vi "quiz3.vi"() -> ()   [LabVIEW 2017]
uses:
  <vilib>/Utility/file.llb/Read Delimited Spreadsheet (string).vi
panel:
  in  "stop 2":bool
  in  "stop":bool
  out "Tab Control 2":T1(tab)
  in  "Contraseña 2":string
  in  "Login 2":string
  in  "Ingresar 2":bool=TRUE
  in  "Ingrese posicion 2":i32
  in  "Usuario a borrar 2":string
  in  "Agregar 2":bool
  in  "Nuevo usuario 2":string
  in  "Nueva contraseña 2":string
  in  "eliminar 2":bool
  in  "Terminar sesion 3":bool
  out "Usuario 2":string
  in  "Terminar sesion 4":bool
  out "leeradd 2":string[][](array[string])
  out "element 4":string
  out "Usuarios y contraseñas 2":string[](array[string])
  out "element 3":i32
  out "Usuarios 2":string[](array[string])
  out "Usuarios":string[](array[string])
  out "element 2":i32
  out "Usuarios y contraseñas":string[](array[string])
  out "leeradd":string[][](array[string])
  out "element":string
  out "Tab Control":T1(tab)
  in  "Contraseña":string
  in  "Login":string
  in  "Ingresar":bool=TRUE
  in  "Ingrese posicion":i32
  in  "Usuario a borrar":string
  in  "Agregar":bool
  in  "Nuevo usuario":string
  in  "Nueva contraseña":string
  in  "eliminar":bool
  in  "Terminar sesion 2":bool
  out "Usuario":string
  in  "Terminar sesion":bool
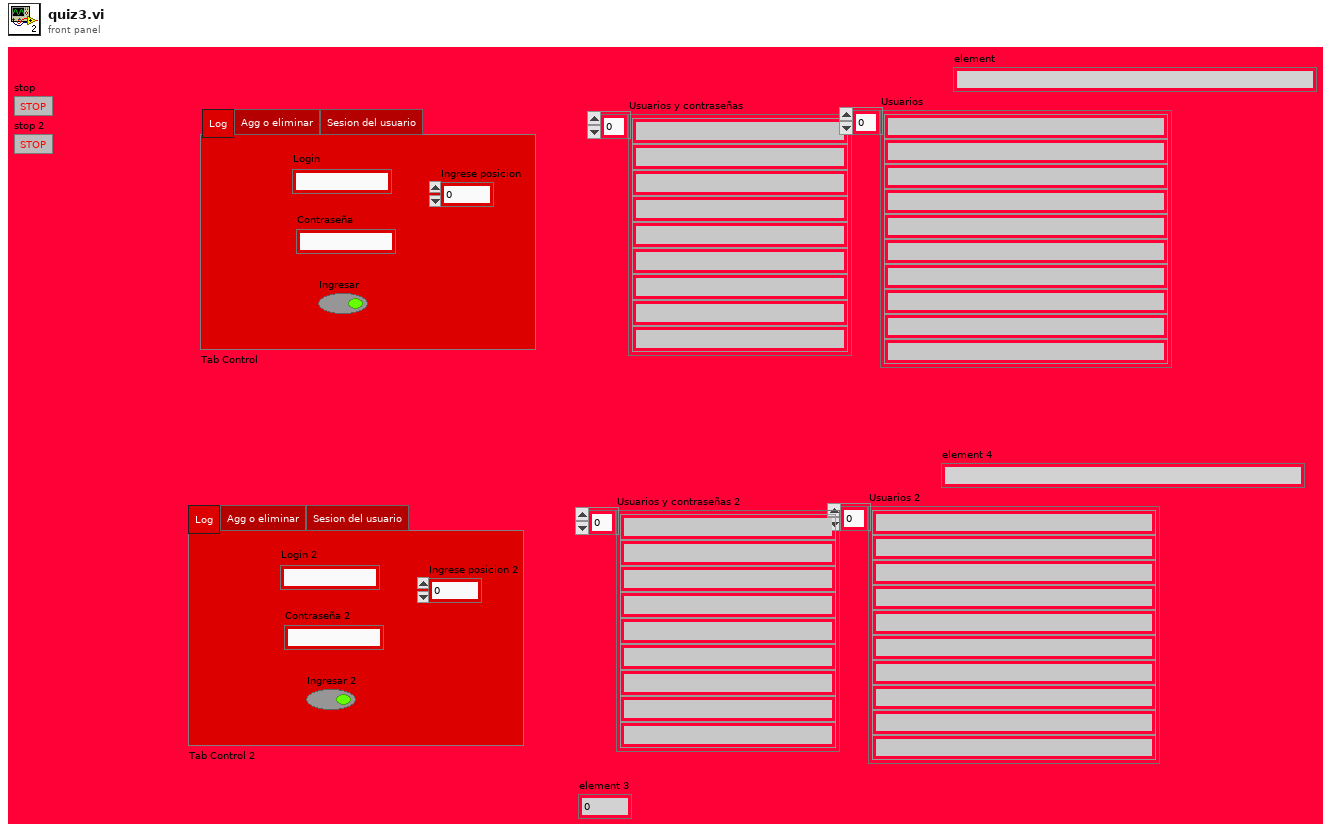
[diagram p1: front panel]
types:
  T1 = enum32{"Log", "Agg o eliminar", "Sesion del usuario"}
  T2 = enum16{"open", "replace", "create", "open or create", "replace or create", "replace or create with confirmation"}
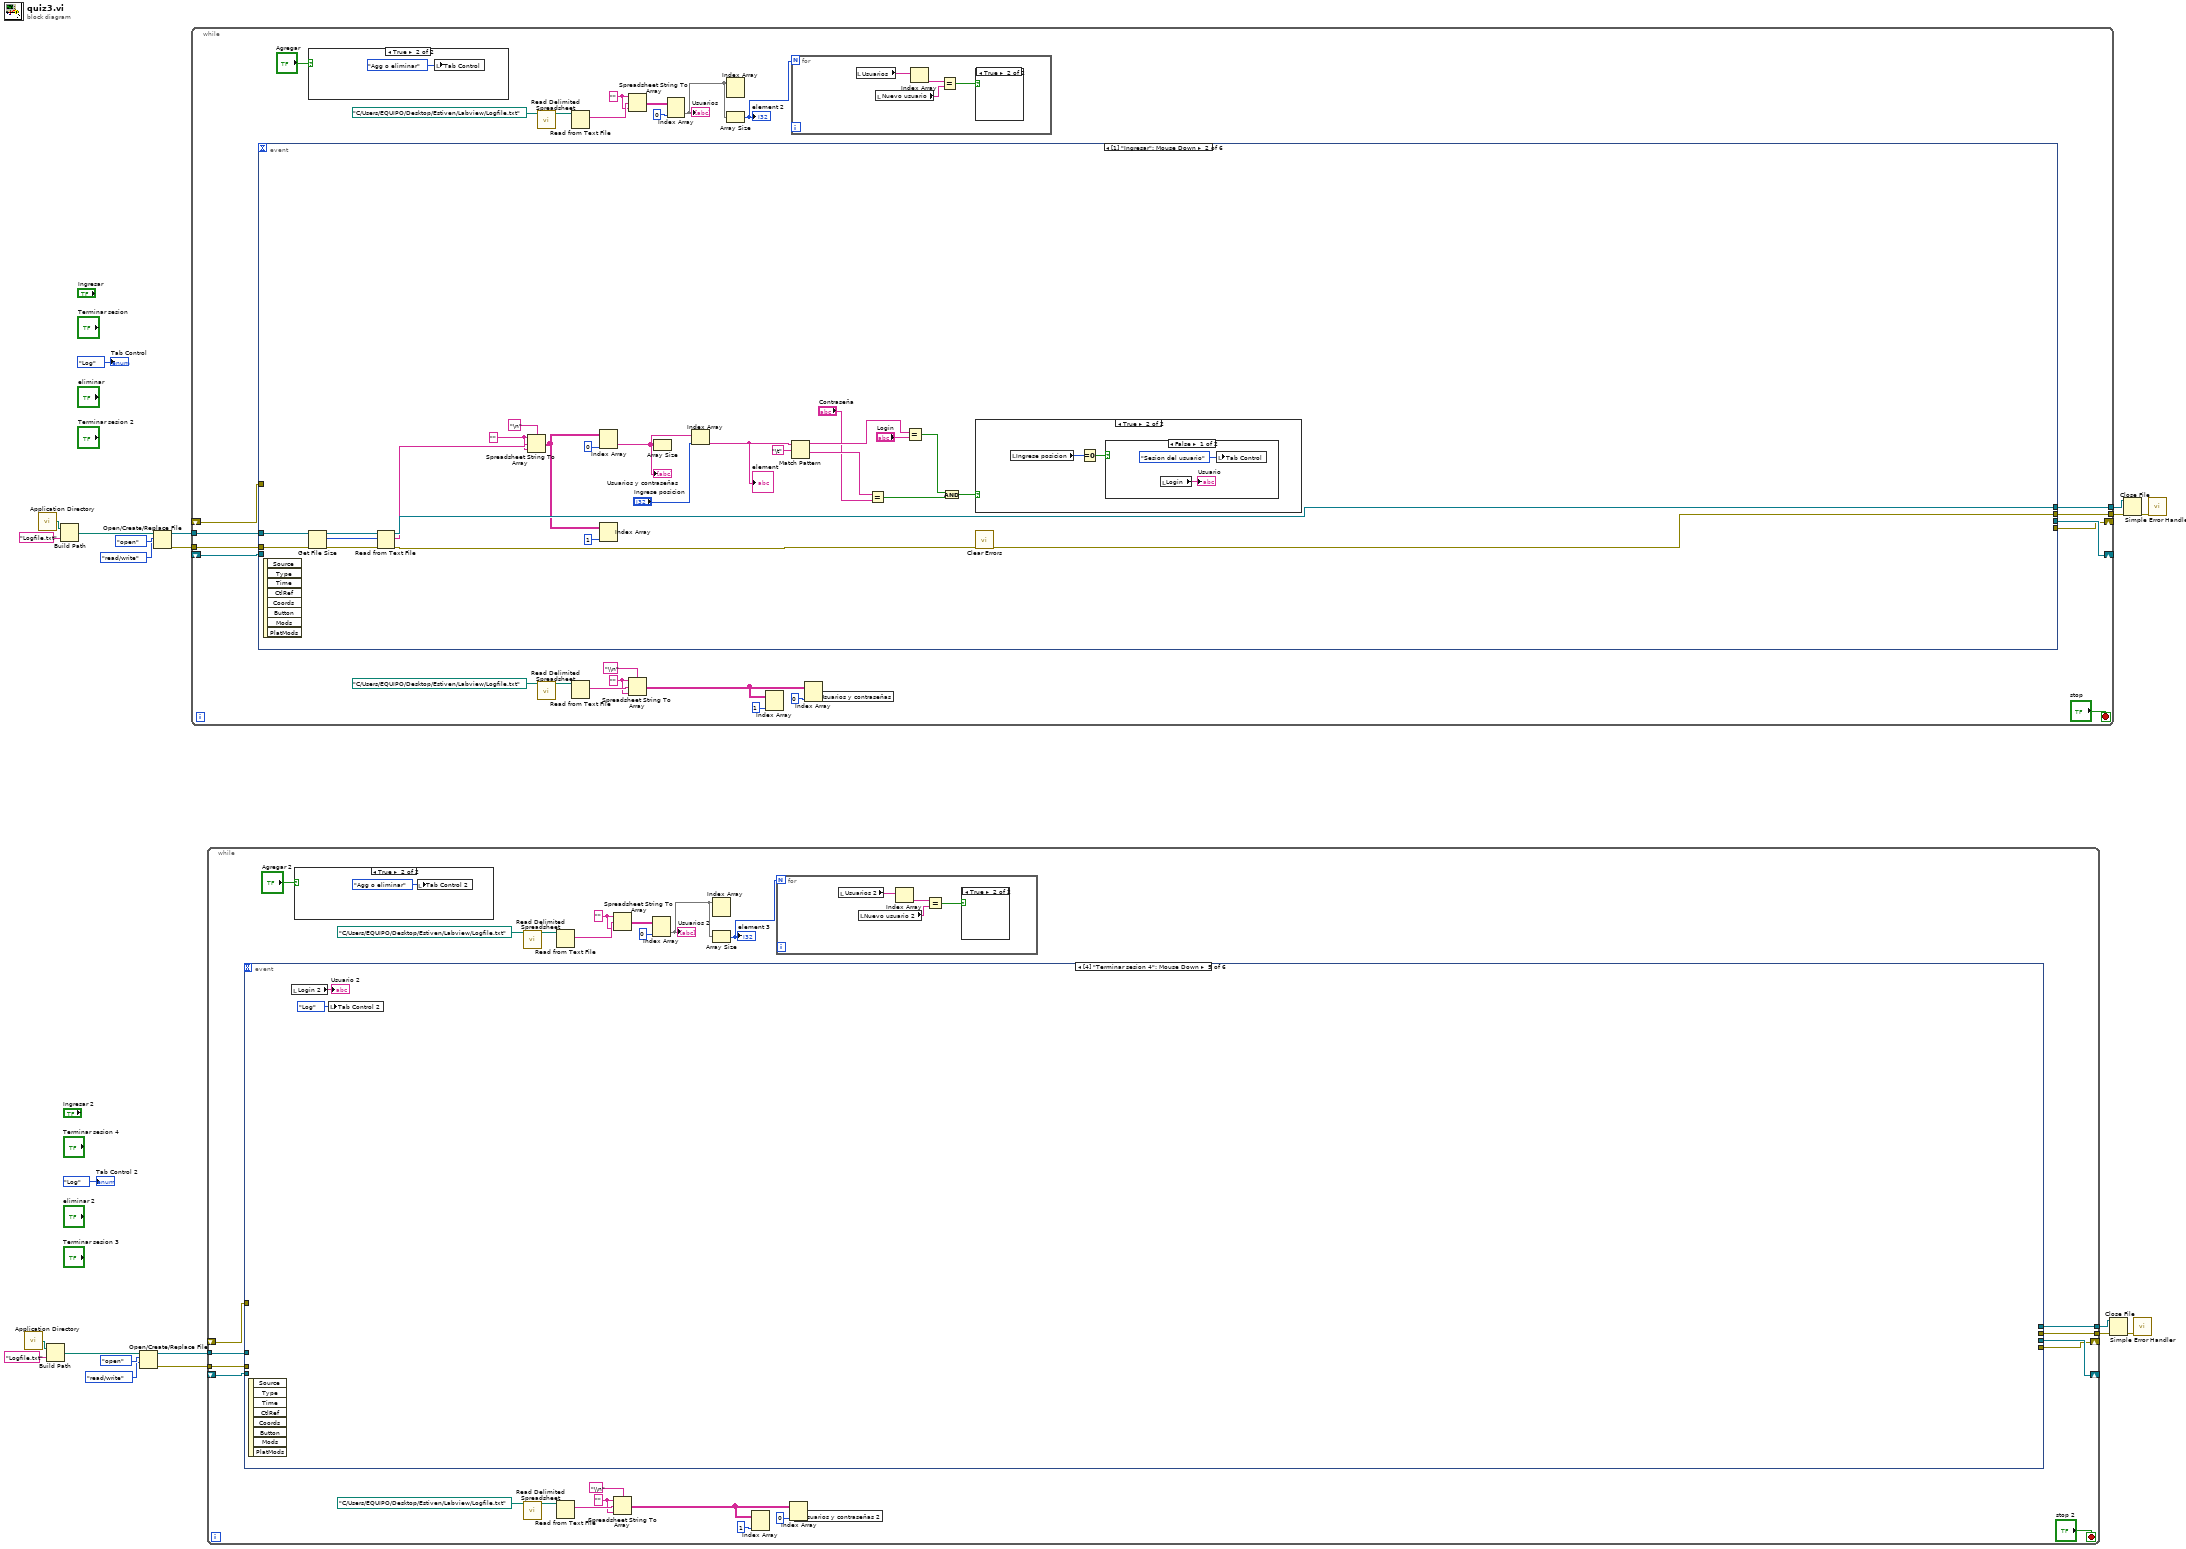
[diagram p0: block diagram]
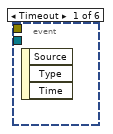
[diagram p4: hidden frame]
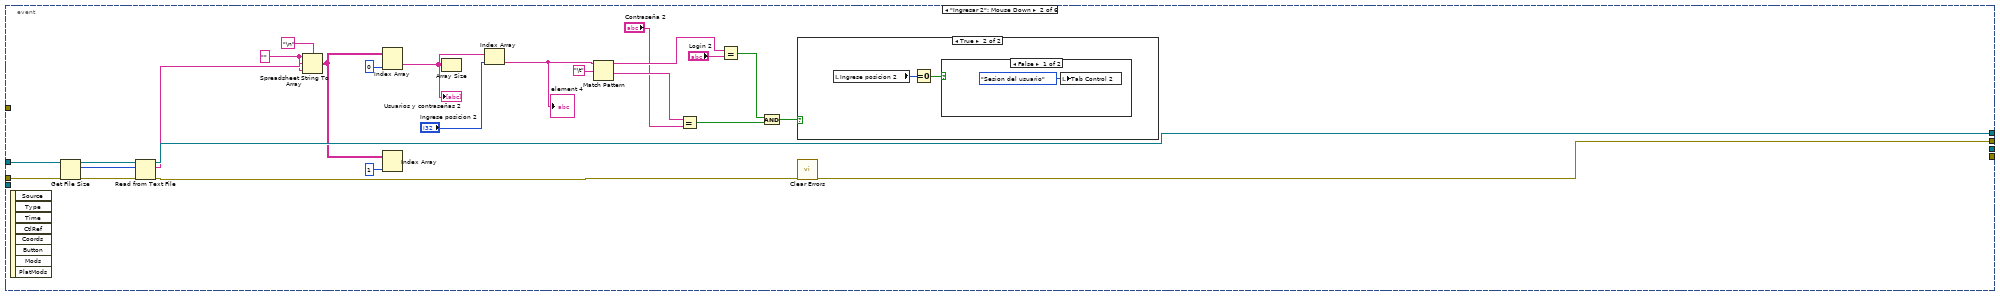
[diagram p5: hidden frame]
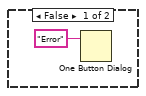
[diagram p6: hidden frame]
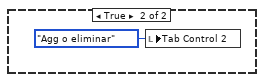
[diagram p7: hidden frame]
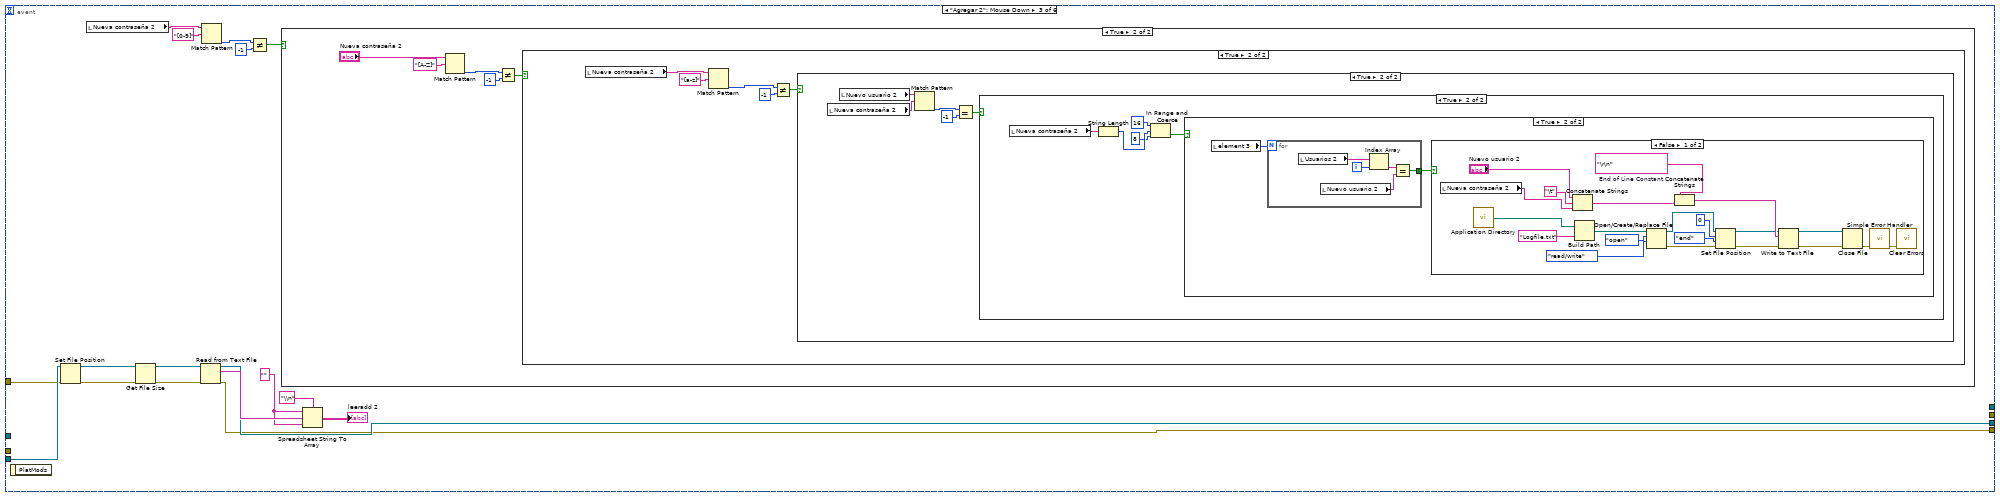
[diagram p8: hidden frame]
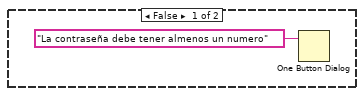
[diagram p9: hidden frame]
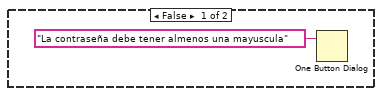
[diagram p10: hidden frame]
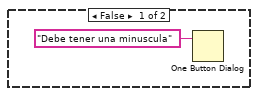
[diagram p11: hidden frame]
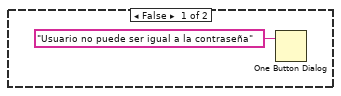
[diagram p12: hidden frame]
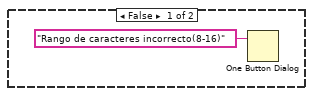
[diagram p13: hidden frame]
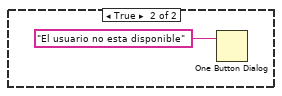
[diagram p14: hidden frame]
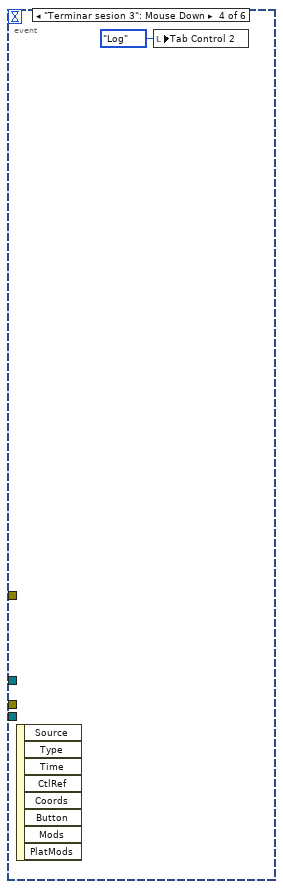
[diagram p15: hidden frame]
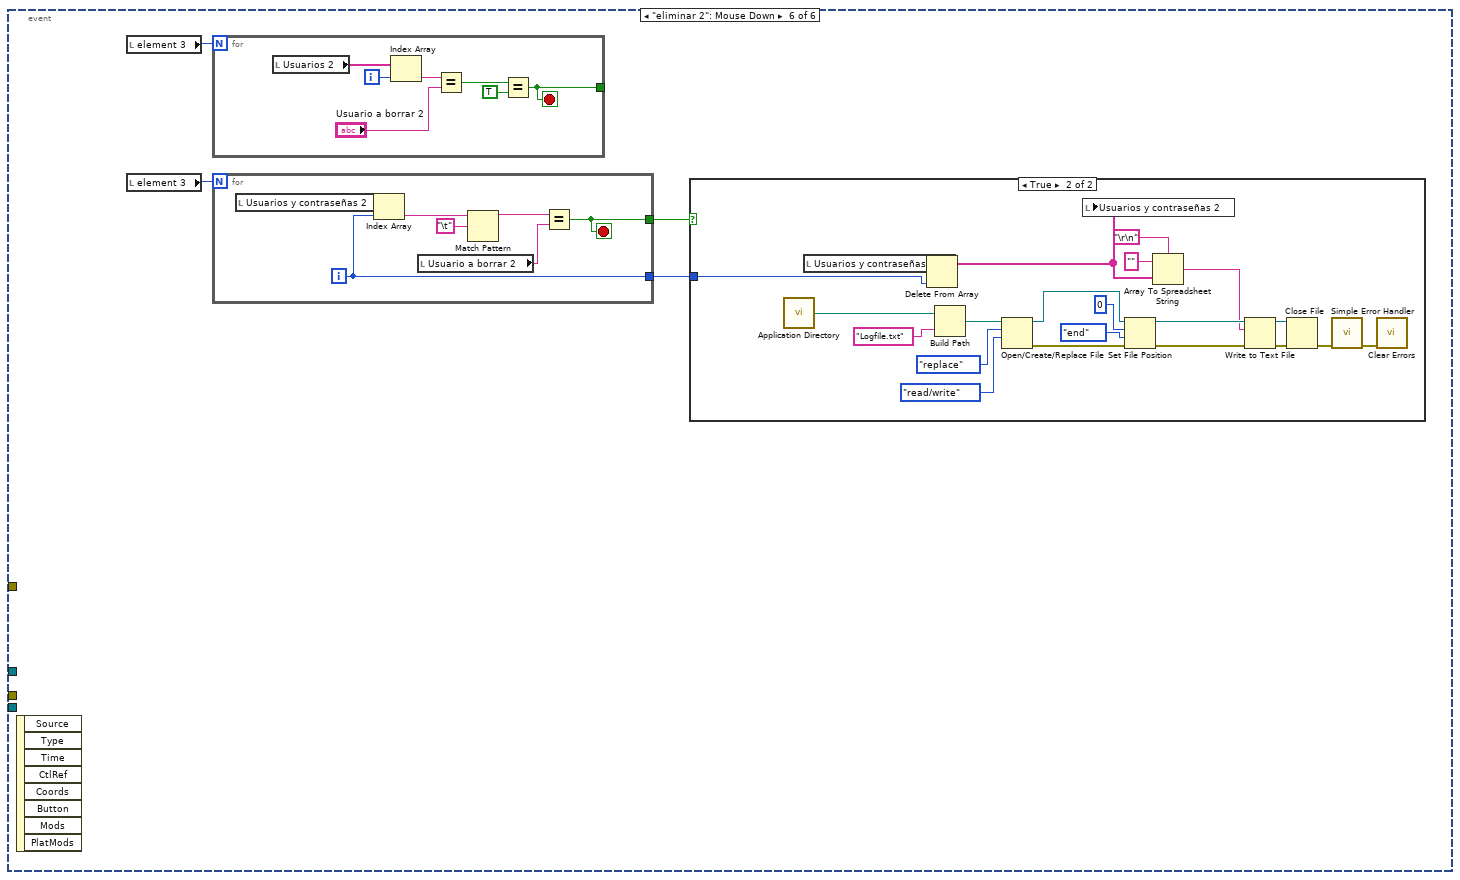
[diagram p16: hidden frame]
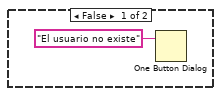
[diagram p17: hidden frame]
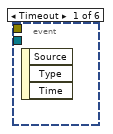
[diagram p20: hidden frame]
diagram:
  n1 = call <vilib>:"Application Directory.vi"() -> ("Application Directory"=w5:path)
  n2 = call <vilib>:"Application Directory.vi"() -> ("Application Directory"=w16:path)
  n3 = Build Path(base path=w5, name or relative path="Logfile.txt") -> (appended path=w6:path)
  n4 = Build Path(base path=w16, name or relative path="Logfile.txt") -> (appended path=w17:path)
  n5 = Open/Create/Replace File(file path (use dialog)=w6, operation (0:open)=T2."open", access (0:read/write)=enum16{"read/write", "read-only", "write-only"}."read/write") -> (refnum out=w8:refnum<file>, error out=w11:errorcluster)  [unwired: 3 in, 1 out]
  n6 = Open/Create/Replace File(file path (use dialog)=w17, operation (0:open)=T2."open", access (0:read/write)=enum16{"read/write", "read-only", "write-only"}."read/write") -> (refnum out=w19:refnum<file>, error out=w22:errorcluster)  [unwired: 3 in, 1 out]
  n7 = while {
    tunnel: w22 -> [w45]
    tunnel: [w49] -> w21
    tunnel: w19 -> [w48]
    tunnel: [w47] -> w18
    shift-right: [w42] -> _
    shift-left: _ -> [w44]
    shift-right: [w41] -> _
    shift-left: _ -> [w43]
    stop <- "stop" stop-if-true
    w26 = "" ("format string")
    w36 = "" ("format string")
    n8 = event shown="[1] \"Ingresar\": Mouse Down" {
      selector: _ -> [_ _ _ _ _ _]
      dyn-events: _ -> [_ _ _ _ _ _]
      timeout: _ -> [_ _ _ _ _ _]
      tunnel: w45 -> [_ w71 _ _ _ _]
      tunnel: [_ w78 _ _ _ _] -> w49
      tunnel: w48 -> [_ w72 _ _ _ _]
      tunnel: [_ w74 _ _ _ _] -> w47
      tunnel: w44 -> [_ _ w90 _ _ _]
      tunnel: w43 -> [_ _ w89 _ _ _]
      tunnel: [_ _ w87 _ _ _] -> w42
      tunnel: [_ _ w86 _ _ _] -> w41
      event Timeout {
        n9 = event-data() -> ()  [unwired: 1 in, 3 out]
      }
      event "Ingresar": Mouse Down {
        w64 = "" ("format string")
        n10 = event-data() -> ()  [unwired: 1 in, 8 out]
        n11 = Get File Size(file=w72, error in=w71) -> (refnum out=w70:refnum<file>, size (in bytes)=w69:i64, 0:w68:errorcluster)
        n12 = Read from Text File(file (use dialog)=w70, count=w69, error in=w68) -> (refnum out=w74:refnum<file>, text=w65:string, error out=w79:errorcluster)  [unwired: 1 in, 1 out]
        n13 = Spreadsheet String To Array(delimiter (Tab)="\n", format string=w64, spreadsheet string=w65, array type (2D Dbl)=w64) -> (array=w63:string[][])
        n14 = Index Array "Index Array"(array=w63, index (col)=0 ("disabled index (col)")) -> (element=w55:string[])  [unwired: 1 in]
        "Usuarios y contraseñas" <- w55
        n15 = Index Array "Index Array"(array=w63, index (col)=1 ("disabled index (col)")) -> ()  [unwired: 1 in, 1 out]
        n16 = Array Size(array=w55) -> ()  [unwired: 1 out]
        n17 = Index Array "Index Array"(array=w55, index="Ingrese posicion") -> (element=w56:string)
        "element" <- w56
        n18 = Match Pattern(string=w56, regular expression="\t") -> (before substring=w67:string, after substring=w66:string)  [unwired: 1 in, 2 out]
        n19 = Equal?(x=w66, y="Contraseña") -> (x = y?=w76:bool)
        n20 = Equal?(x=w67, y="Login") -> (x = y?=w77:bool)
        n21 = And(x=w77, y=w76) -> (x .and. y?=w75:bool)
        n22 = case shown="True" w75 {
          frame False {
            n23 = One Button Dialog(message="Error") -> ()  [unwired: 1 in, 1 out]
          }
          frame True {
            n24 = local read "Ingrese posicion"() -> (w82:i32)
            n25 = Equal To 0?(x=w82) -> (x = 0?=w81:bool)
            n26 = case shown="False" w81 {
              frame False {
                n27 = local read "Login"() -> (→"Usuario":string)
                n28 = local write "Tab Control"(T1."Sesion del usuario" ("Tab Control")) -> ()
              }
              frame True {
                n29 = local write "Tab Control"(enum32{"Log", "Agg o eliminar"}."Agg o eliminar" ("Tab Control")) -> ()
              }
            }
          }
        }
        n30 = call <vilib>:"Clear Errors.vi"("error in (no error)"=w79) -> ("error out"=w78:errorcluster)  [unwired: 5 in, 1 out]
      }
      event "Agregar": Mouse Down {
        w91 = "" ("format string")
        n31 = event-data() -> ()  [unwired: 1 in, 1 out]
        n32 = Set File Position(refnum=w90, error in=w89) -> (refnum out=w97:refnum<file>, error out=w94:errorcluster)  [unwired: 2 in]
        n33 = local read "Nueva contraseña"() -> (w102:string)
        n34 = Get File Size(file=w97, error in=w94) -> (refnum out=w96:refnum<file>, 0:w93:errorcluster)  [unwired: 1 out]
        n35 = Read from Text File(file (use dialog)=w96, error in=w93) -> (refnum out=w87:refnum<file>, text=w95:string, error out=w86:errorcluster)  [unwired: 2 in, 1 out]
        n36 = Match Pattern(string=w102, regular expression="[0-9]") -> (offset past match=w100:i32)  [unwired: 1 in, 3 out]
        n37 = Not Equal?(x=w100, y=-1) -> (x != y?=w98:bool)
        n38 = case shown="True" w98 {
          frame False {
            n39 = One Button Dialog(message="La contraseña debe tener almenos un numero") -> ()  [unwired: 1 in, 1 out]
          }
          frame True {
            n40 = Match Pattern(string="Nueva contraseña", regular expression="[A-Z]") -> (offset past match=w107:i32)  [unwired: 1 in, 3 out]
            n41 = Not Equal?(x=w107, y=-1) -> (x != y?=w104:bool)
            n42 = case shown="True" w104 {
              frame False {
                n43 = One Button Dialog(message="La contraseña debe tener almenos una mayuscula") -> ()  [unwired: 1 in, 1 out]
              }
              frame True {
                n44 = local read "Nueva contraseña"() -> (w111:string)
                n45 = Match Pattern(string=w111, regular expression="[a-z]") -> (offset past match=w113:i32)  [unwired: 1 in, 3 out]
                n46 = Not Equal?(x=w113, y=-1) -> (x != y?=w110:bool)
                n47 = case shown="True" w110 {
                  frame False {
                    n48 = One Button Dialog(message="Debe tener una minuscula") -> ()  [unwired: 1 in, 1 out]
                  }
                  frame True {
                    n49 = local read "Nueva contraseña"() -> (w120:string)
                    n50 = local read "Nuevo usuario"() -> (w119:string)
                    n51 = Match Pattern(string=w119, regular expression=w120) -> (offset past match=w118:i32)  [unwired: 1 in, 3 out]
                    n52 = Equal?(x=w118, y=-1) -> (x = y?=w117:bool)
                    n53 = case shown="True" w117 {
                      frame False {
                        n54 = One Button Dialog(message="Usuario no puede ser igual a la contraseña") -> ()  [unwired: 1 in, 1 out]
                      }
                      frame True {
                        n55 = local read "Nueva contraseña"() -> (w126:string)
                        n56 = String Length(string=w126) -> (length=w125:i32)
                        n57 = In Range and Coerce(upper limit=16, x=w125, lower limit=8) -> (In Range?=w122:bool)  [unwired: 1 out]
                        n58 = case shown="True" w122 {
                          frame False {
                            n59 = One Button Dialog(message="Rango de caracteres incorrecto(8-16)") -> ()  [unwired: 1 in, 1 out]
                          }
                          frame True {
                            n60 = local read "element 2"() -> (w129:i32)
                            n61 = for {
                              N: w129 -> [_]
                              tunnel: [w154] -> w128
                              i -> [w152]
                              n62 = local read "Usuarios"() -> (w153:string[])
                              n63 = local read "Nuevo usuario"() -> (w156:string)
                              n64 = Index Array(array=w153, index=w152) -> (element=w155:string)
                              n65 = Equal?(x=w155, y=w156) -> (x = y?=w154:bool)
                            }
                            n66 = case shown="False" w128 {
                              frame False {
                                w136 = "\r\n"  # End of Line Constant
                                n67 = local read "Nueva contraseña"() -> (w137:string)
                                n68 = call <vilib>:"Application Directory.vi"() -> ("Application Directory"=w139:path)
                                n69 = Concatenate Strings "Concatenate Strings"("Nuevo usuario", "\t", w137) -> (w150:string)
                                n70 = Build Path(base path=w139, name or relative path="Logfile.txt") -> (appended path=w140:path)
                                n71 = Open/Create/Replace File(file path (use dialog)=w140, operation (0:open)=T2."open", access (0:read/write)=enum16{"read/write", "read-only", "write-only"}."read/write") -> (refnum out=w141:refnum<file>, error out=w144:errorcluster)  [unwired: 3 in, 1 out]
                                n72 = Concatenate Strings "Concatenate Strings"(w136, w150) -> (w149:string)
                                n73 = Set File Position(offset (in bytes) (0)=i64 0, refnum=w141, from (0:start)=enum16{"start", "end", "current"}."end", error in=w144) -> (refnum out=w142:refnum<file>, error out=w145:errorcluster)
                                n74 = Write to Text File(file (use dialog)=w142, text=w149, error in=w145) -> (refnum out=w143:refnum<file>, error out=w146:errorcluster)  [unwired: 1 in, 1 out]
                                n75 = Close File(refnum=w143, error in=w146) -> (error out=w147:errorcluster)  [unwired: 1 out]
                                n76 = call <vilib>:"Simple Error Handler.vi"("error in (no error)"=w147) -> ("error out"=w148:errorcluster)  [unwired: 4 in, 4 out]
                                n77 = call <vilib>:"Clear Errors.vi"("error in (no error)"=w148) -> ()  [unwired: 5 in, 2 out]
                              }
                              frame True {
                                n78 = One Button Dialog(message="El usuario no esta disponible") -> ()  [unwired: 1 in, 1 out]
                              }
                            }
                          }
                        }
                      }
                    }
                  }
                }
              }
            }
          }
        }
        n79 = Spreadsheet String To Array(delimiter (Tab)="\\n", format string=w91, spreadsheet string=w95, array type (2D Dbl)=w91) -> (array=→"leeradd":string[][])
      }
      event "Terminar sesion 2": Mouse Down {
        n80 = event-data() -> ()  [unwired: 1 in, 8 out]
        n81 = local write "Tab Control"(T1."Log" ("Tab Control")) -> ()
      }
      event "Terminar sesion": Mouse Down {
        n82 = event-data() -> ()  [unwired: 1 in, 8 out]
        n83 = local write "Tab Control"(T1."Log" ("Tab Control")) -> ()
      }
      event "eliminar": Mouse Down {
        n84 = event-data() -> ()  [unwired: 1 in, 8 out]
        n85 = local read "element 2"() -> (w162:i32)
        n86 = local read "element 2"() -> (w161:i32)
        n87 = for {
          N: w162 -> [_]
          tunnel: [w171] -> _
          i -> [w170]
          stop <- w171 stop-if-true
          n88 = local read "Usuarios"() -> (w173:string[])
          n89 = Index Array(array=w173, index=w170) -> (element=w172:string)
          n90 = Equal?(x=w172, y="Usuario a borrar") -> (x = y?=w176:bool)
          n91 = Equal?(x=w176, y=TRUE) -> (x = y?=w171:bool)
        }
        n92 = for {
          N: w161 -> [_]
          tunnel: [w165] -> w159
          tunnel: [w163] -> w160
          i -> [w163]
          stop <- w165 stop-if-true
          n93 = local read "Usuarios y contraseñas"() -> (w164:string[])
          n94 = Index Array(array=w164, index=w163) -> (element=w169:string)
          n95 = local read "Usuario a borrar"() -> (w166:string)
          n96 = Match Pattern(string=w169, regular expression="\t") -> (before substring=w167:string)  [unwired: 1 in, 3 out]
          n97 = Equal?(x=w167, y=w166) -> (x = y?=w165:bool)
        }
        n98 = case shown="True" w159 {
          tunnel: w160 -> [_ w183]
          frame False {
            n99 = One Button Dialog(message="El usuario no existe") -> ()  [unwired: 1 in, 1 out]
          }
          frame True {
            n100 = call <vilib>:"Application Directory.vi"() -> ("Application Directory"=w189:path)
            n101 = local read "Usuarios y contraseñas"() -> (w182:string[])
            n102 = Delete From Array "Delete From Array"(array=w182, index=w183) -> (array with subset deleted=w180:string[])  [unwired: 1 in, 1 out]
            n103 = Build Path(base path=w189, name or relative path="Logfile.txt") -> (appended path=w190:path)
            n104 = Open/Create/Replace File(file path (use dialog)=w190, operation (0:open)=T2."replace", access (0:read/write)=enum16{"read/write", "read-only", "write-only"}."read/write") -> (refnum out=w191:refnum<file>, error out=w194:errorcluster)  [unwired: 3 in, 1 out]
            n105 = local write "Usuarios y contraseñas"(w180) -> ()
            n106 = Set File Position(offset (in bytes) (0)=i64 0, refnum=w191, from (0:start)=enum16{"start", "end", "current"}."end", error in=w194) -> (refnum out=w192:refnum<file>, error out=w195:errorcluster)
            n107 = Array To Spreadsheet String(delimiter (Tab)="\r\n", array=w180, 3:"" ("format string")) -> (spreadsheet string=w179:string)
            n108 = Write to Text File(file (use dialog)=w192, text=w179, error in=w195) -> (refnum out=w193:refnum<file>, error out=w196:errorcluster)  [unwired: 1 in, 1 out]
            n109 = Close File(refnum=w193, error in=w196) -> (error out=w197:errorcluster)  [unwired: 1 out]
            n110 = call <vilib>:"Simple Error Handler.vi"("error in (no error)"=w197) -> ("error out"=w198:errorcluster)  [unwired: 4 in, 4 out]
            n111 = call <vilib>:"Clear Errors.vi"("error in (no error)"=w198) -> ()  [unwired: 5 in, 2 out]
          }
        }
      }
    }
    n112 = case shown="True" "Agregar" {
      frame False {
      }
      frame True {
        n113 = local write "Tab Control"(T1."Agg o eliminar" ("Tab Control")) -> ()
      }
    }
    n114 = call-poly <vilib>:"Read Delimited Spreadsheet.vi"("file path (dialog if empty)"=path "C:/Users/EQUIPO/Desktop/Estiven/Labview/Logfile.txt") -> ("new file path (Not A Path if cancelled)"=w37:path)  [unwired: 9 in, 5 out]
    n115 = call-poly <vilib>:"Read Delimited Spreadsheet.vi"("file path (dialog if empty)"=path "C:/Users/EQUIPO/Desktop/Estiven/Labview/Logfile.txt") -> ("new file path (Not A Path if cancelled)"=w32:path)  [unwired: 9 in, 5 out]
    n116 = Read from Text File(file (use dialog)=w37) -> (text=w38:string)  [unwired: 3 in, 3 out]
    n117 = Read from Text File(file (use dialog)=w32) -> (text=w31:string)  [unwired: 3 in, 3 out]
    n118 = Spreadsheet String To Array(format string=w36, spreadsheet string=w38, array type (2D Dbl)=w36) -> (array=w39:string[][])  [unwired: 1 in]
    n119 = Spreadsheet String To Array(delimiter (Tab)="\\n", format string=w26, spreadsheet string=w31, array type (2D Dbl)=w26) -> (array=w30:string[][])
    n120 = Index Array(array=w39, index (col)=0 ("index")) -> (element=w33:string[])  [unwired: 1 in]
    "Usuarios" <- w33
    n121 = Index Array "Index Array"(array=w33) -> ()  [unwired: 2 in, 2 out]
    n122 = Array Size(array=w33) -> (size(s)=w40:i32)
    "element 2" <- w40
    n123 = Index Array(array=w30, index (col)=1 ("disabled index (col)")) -> ()  [unwired: 1 in, 1 out]
    n124 = for {
      N: w40 -> [_]
      n125 = local read "Usuarios"() -> (w53:string[])
      n126 = local read "Nuevo usuario"() -> (w51:string)
      n127 = Index Array(array=w53) -> (element=w52:string)  [unwired: 1 in]
      n128 = Equal?(x=w52, y=w51) -> (x = y?=w50:bool)
      n129 = case shown="True" w50 {
        frame False {
        }
        frame True {
        }
      }
    }
    n130 = Index Array(array=w30, index (col)=0 ("index")) -> (element=w29:string[])  [unwired: 1 in]
    n131 = local write "Usuarios y contraseñas"(w29) -> ()
  }
  n132 = while {
    tunnel: w11 -> [w221]
    tunnel: [w225] -> w10
    tunnel: w8 -> [w224]
    tunnel: [w223] -> w7
    shift-right: [w218] -> _
    shift-left: _ -> [w220]
    shift-right: [w217] -> _
    shift-left: _ -> [w219]
    stop <- "stop 2" stop-if-true
    w202 = "" ("format string")
    w212 = "" ("format string")
    n133 = event shown="[4] \"Terminar sesion 4\": Mouse Down" {
      selector: _ -> [_ _ _ _ _ _]
      dyn-events: _ -> [_ _ _ _ _ _]
      timeout: _ -> [_ _ _ _ _ _]
      tunnel: w221 -> [_ w247 _ _ _ _]
      tunnel: [_ w254 _ _ _ _] -> w225
      tunnel: w224 -> [_ w248 _ _ _ _]
      tunnel: [_ w250 _ _ _ _] -> w223
      tunnel: w220 -> [_ _ w265 _ _ _]
      tunnel: w219 -> [_ _ w264 _ _ _]
      tunnel: [_ _ w262 _ _ _] -> w218
      tunnel: [_ _ w261 _ _ _] -> w217
      event Timeout {
        n134 = event-data() -> ()  [unwired: 1 in, 3 out]
      }
      event "Ingresar 2": Mouse Down {
        w240 = "" ("format string")
        n135 = event-data() -> ()  [unwired: 1 in, 8 out]
        n136 = Get File Size(file=w248, error in=w247) -> (refnum out=w246:refnum<file>, size (in bytes)=w245:i64, 0:w244:errorcluster)
        n137 = Read from Text File(file (use dialog)=w246, count=w245, error in=w244) -> (refnum out=w250:refnum<file>, text=w241:string, error out=w255:errorcluster)  [unwired: 1 in, 1 out]
        n138 = Spreadsheet String To Array(delimiter (Tab)="\n", format string=w240, spreadsheet string=w241, array type (2D Dbl)=w240) -> (array=w239:string[][])
        n139 = Index Array "Index Array"(array=w239, index (col)=0 ("disabled index (col)")) -> (element=w231:string[])  [unwired: 1 in]
        "Usuarios y contraseñas 2" <- w231
        n140 = Index Array "Index Array"(array=w239, index (col)=1 ("disabled index (col)")) -> ()  [unwired: 1 in, 1 out]
        n141 = Array Size(array=w231) -> ()  [unwired: 1 out]
        n142 = Index Array "Index Array"(array=w231, index="Ingrese posicion 2") -> (element=w232:string)
        "element 4" <- w232
        n143 = Match Pattern(string=w232, regular expression="\t") -> (before substring=w243:string, after substring=w242:string)  [unwired: 1 in, 2 out]
        n144 = Equal?(x=w242, y="Contraseña 2") -> (x = y?=w252:bool)
        n145 = Equal?(x=w243, y="Login 2") -> (x = y?=w253:bool)
        n146 = And(x=w253, y=w252) -> (x .and. y?=w251:bool)
        n147 = case shown="True" w251 {
          frame False {
            n148 = One Button Dialog(message="Error") -> ()  [unwired: 1 in, 1 out]
          }
          frame True {
            n149 = local read "Ingrese posicion 2"() -> (w258:i32)
            n150 = Equal To 0?(x=w258) -> (x = 0?=w257:bool)
            n151 = case shown="False" w257 {
              frame False {
                n152 = local write "Tab Control 2"(T1."Sesion del usuario" ("Tab Control")) -> ()
              }
              frame True {
                n153 = local write "Tab Control 2"(enum32{"Log", "Agg o eliminar"}."Agg o eliminar" ("Tab Control")) -> ()
              }
            }
          }
        }
        n154 = call <vilib>:"Clear Errors.vi"("error in (no error)"=w255) -> ("error out"=w254:errorcluster)  [unwired: 5 in, 1 out]
      }
      event "Agregar 2": Mouse Down {
        w266 = "" ("format string")
        n155 = event-data() -> ()  [unwired: 1 in, 1 out]
        n156 = Set File Position(refnum=w265, error in=w264) -> (refnum out=w272:refnum<file>, error out=w269:errorcluster)  [unwired: 2 in]
        n157 = local read "Nueva contraseña 2"() -> (w277:string)
        n158 = Get File Size(file=w272, error in=w269) -> (refnum out=w271:refnum<file>, 0:w268:errorcluster)  [unwired: 1 out]
        n159 = Read from Text File(file (use dialog)=w271, error in=w268) -> (refnum out=w262:refnum<file>, text=w270:string, error out=w261:errorcluster)  [unwired: 2 in, 1 out]
        n160 = Match Pattern(string=w277, regular expression="[0-9]") -> (offset past match=w275:i32)  [unwired: 1 in, 3 out]
        n161 = Not Equal?(x=w275, y=-1) -> (x != y?=w273:bool)
        n162 = case shown="True" w273 {
          frame False {
            n163 = One Button Dialog(message="La contraseña debe tener almenos un numero") -> ()  [unwired: 1 in, 1 out]
          }
          frame True {
            n164 = Match Pattern(string="Nueva contraseña 2", regular expression="[A-Z]") -> (offset past match=w282:i32)  [unwired: 1 in, 3 out]
            n165 = Not Equal?(x=w282, y=-1) -> (x != y?=w279:bool)
            n166 = case shown="True" w279 {
              frame False {
                n167 = One Button Dialog(message="La contraseña debe tener almenos una mayuscula") -> ()  [unwired: 1 in, 1 out]
              }
              frame True {
                n168 = local read "Nueva contraseña 2"() -> (w286:string)
                n169 = Match Pattern(string=w286, regular expression="[a-z]") -> (offset past match=w288:i32)  [unwired: 1 in, 3 out]
                n170 = Not Equal?(x=w288, y=-1) -> (x != y?=w285:bool)
                n171 = case shown="True" w285 {
                  frame False {
                    n172 = One Button Dialog(message="Debe tener una minuscula") -> ()  [unwired: 1 in, 1 out]
                  }
                  frame True {
                    n173 = local read "Nueva contraseña 2"() -> (w295:string)
                    n174 = local read "Nuevo usuario 2"() -> (w294:string)
                    n175 = Match Pattern(string=w294, regular expression=w295) -> (offset past match=w293:i32)  [unwired: 1 in, 3 out]
                    n176 = Equal?(x=w293, y=-1) -> (x = y?=w292:bool)
                    n177 = case shown="True" w292 {
                      frame False {
                        n178 = One Button Dialog(message="Usuario no puede ser igual a la contraseña") -> ()  [unwired: 1 in, 1 out]
                      }
                      frame True {
                        n179 = local read "Nueva contraseña 2"() -> (w301:string)
                        n180 = String Length(string=w301) -> (length=w300:i32)
                        n181 = In Range and Coerce(upper limit=16, x=w300, lower limit=8) -> (In Range?=w297:bool)  [unwired: 1 out]
                        n182 = case shown="True" w297 {
                          frame False {
                            n183 = One Button Dialog(message="Rango de caracteres incorrecto(8-16)") -> ()  [unwired: 1 in, 1 out]
                          }
                          frame True {
                            n184 = local read "element 3"() -> (w304:i32)
                            n185 = for {
                              N: w304 -> [_]
                              tunnel: [w329] -> w303
                              i -> [w327]
                              n186 = local read "Usuarios 2"() -> (w328:string[])
                              n187 = local read "Nuevo usuario 2"() -> (w331:string)
                              n188 = Index Array(array=w328, index=w327) -> (element=w330:string)
                              n189 = Equal?(x=w330, y=w331) -> (x = y?=w329:bool)
                            }
                            n190 = case shown="False" w303 {
                              frame False {
                                w311 = "\r\n"  # End of Line Constant
                                n191 = local read "Nueva contraseña 2"() -> (w312:string)
                                n192 = call <vilib>:"Application Directory.vi"() -> ("Application Directory"=w314:path)
                                n193 = Concatenate Strings "Concatenate Strings"("Nuevo usuario 2", "\t", w312) -> (w325:string)
                                n194 = Build Path(base path=w314, name or relative path="Logfile.txt") -> (appended path=w315:path)
                                n195 = Open/Create/Replace File(file path (use dialog)=w315, operation (0:open)=T2."open", access (0:read/write)=enum16{"read/write", "read-only", "write-only"}."read/write") -> (refnum out=w316:refnum<file>, error out=w319:errorcluster)  [unwired: 3 in, 1 out]
                                n196 = Concatenate Strings "Concatenate Strings"(w311, w325) -> (w324:string)
                                n197 = Set File Position(offset (in bytes) (0)=i64 0, refnum=w316, from (0:start)=enum16{"start", "end", "current"}."end", error in=w319) -> (refnum out=w317:refnum<file>, error out=w320:errorcluster)
                                n198 = Write to Text File(file (use dialog)=w317, text=w324, error in=w320) -> (refnum out=w318:refnum<file>, error out=w321:errorcluster)  [unwired: 1 in, 1 out]
                                n199 = Close File(refnum=w318, error in=w321) -> (error out=w322:errorcluster)  [unwired: 1 out]
                                n200 = call <vilib>:"Simple Error Handler.vi"("error in (no error)"=w322) -> ("error out"=w323:errorcluster)  [unwired: 4 in, 4 out]
                                n201 = call <vilib>:"Clear Errors.vi"("error in (no error)"=w323) -> ()  [unwired: 5 in, 2 out]
                              }
                              frame True {
                                n202 = One Button Dialog(message="El usuario no esta disponible") -> ()  [unwired: 1 in, 1 out]
                              }
                            }
                          }
                        }
                      }
                    }
                  }
                }
              }
            }
          }
        }
        n203 = Spreadsheet String To Array(delimiter (Tab)="\\n", format string=w266, spreadsheet string=w270, array type (2D Dbl)=w266) -> (array=→"leeradd 2":string[][])
      }
      event "Terminar sesion 3": Mouse Down {
        n204 = event-data() -> ()  [unwired: 1 in, 8 out]
        n205 = local write "Tab Control 2"(T1."Log" ("Tab Control")) -> ()
      }
      event "Terminar sesion 4": Mouse Down {
        n206 = event-data() -> ()  [unwired: 1 in, 8 out]
        n207 = local read "Login 2"() -> (→"Usuario 2":string)
        n208 = local write "Tab Control 2"(T1."Log" ("Tab Control")) -> ()
      }
      event "eliminar 2": Mouse Down {
        n209 = event-data() -> ()  [unwired: 1 in, 8 out]
        n210 = local read "element 3"() -> (w338:i32)
        n211 = local read "element 3"() -> (w337:i32)
        n212 = for {
          N: w338 -> [_]
          tunnel: [w347] -> _
          i -> [w346]
          stop <- w347 stop-if-true
          n213 = local read "Usuarios 2"() -> (w349:string[])
          n214 = Index Array(array=w349, index=w346) -> (element=w348:string)
          n215 = Equal?(x=w348, y="Usuario a borrar 2") -> (x = y?=w352:bool)
          n216 = Equal?(x=w352, y=TRUE) -> (x = y?=w347:bool)
        }
        n217 = for {
          N: w337 -> [_]
          tunnel: [w341] -> w335
          tunnel: [w339] -> w336
          i -> [w339]
          stop <- w341 stop-if-true
          n218 = local read "Usuarios y contraseñas 2"() -> (w340:string[])
          n219 = Index Array(array=w340, index=w339) -> (element=w345:string)
          n220 = local read "Usuario a borrar 2"() -> (w342:string)
          n221 = Match Pattern(string=w345, regular expression="\t") -> (before substring=w343:string)  [unwired: 1 in, 3 out]
          n222 = Equal?(x=w343, y=w342) -> (x = y?=w341:bool)
        }
        n223 = case shown="True" w335 {
          tunnel: w336 -> [_ w359]
          frame False {
            n224 = One Button Dialog(message="El usuario no existe") -> ()  [unwired: 1 in, 1 out]
          }
          frame True {
            n225 = call <vilib>:"Application Directory.vi"() -> ("Application Directory"=w365:path)
            n226 = local read "Usuarios y contraseñas 2"() -> (w358:string[])
            n227 = Delete From Array "Delete From Array"(array=w358, index=w359) -> (array with subset deleted=w356:string[])  [unwired: 1 in, 1 out]
            n228 = Build Path(base path=w365, name or relative path="Logfile.txt") -> (appended path=w366:path)
            n229 = Open/Create/Replace File(file path (use dialog)=w366, operation (0:open)=T2."replace", access (0:read/write)=enum16{"read/write", "read-only", "write-only"}."read/write") -> (refnum out=w367:refnum<file>, error out=w370:errorcluster)  [unwired: 3 in, 1 out]
            n230 = local write "Usuarios y contraseñas 2"(w356) -> ()
            n231 = Set File Position(offset (in bytes) (0)=i64 0, refnum=w367, from (0:start)=enum16{"start", "end", "current"}."end", error in=w370) -> (refnum out=w368:refnum<file>, error out=w371:errorcluster)
            n232 = Array To Spreadsheet String(delimiter (Tab)="\r\n", array=w356, 3:"" ("format string")) -> (spreadsheet string=w355:string)
            n233 = Write to Text File(file (use dialog)=w368, text=w355, error in=w371) -> (refnum out=w369:refnum<file>, error out=w372:errorcluster)  [unwired: 1 in, 1 out]
            n234 = Close File(refnum=w369, error in=w372) -> (error out=w373:errorcluster)  [unwired: 1 out]
            n235 = call <vilib>:"Simple Error Handler.vi"("error in (no error)"=w373) -> ("error out"=w374:errorcluster)  [unwired: 4 in, 4 out]
            n236 = call <vilib>:"Clear Errors.vi"("error in (no error)"=w374) -> ()  [unwired: 5 in, 2 out]
          }
        }
      }
    }
    n237 = case shown="True" "Agregar 2" {
      frame False {
      }
      frame True {
        n238 = local write "Tab Control 2"(T1."Agg o eliminar" ("Tab Control")) -> ()
      }
    }
    n239 = call-poly <vilib>:"Read Delimited Spreadsheet.vi"("file path (dialog if empty)"=path "C:/Users/EQUIPO/Desktop/Estiven/Labview/Logfile.txt") -> ("new file path (Not A Path if cancelled)"=w213:path)  [unwired: 9 in, 5 out]
    n240 = call-poly <vilib>:"Read Delimited Spreadsheet.vi"("file path (dialog if empty)"=path "C:/Users/EQUIPO/Desktop/Estiven/Labview/Logfile.txt") -> ("new file path (Not A Path if cancelled)"=w208:path)  [unwired: 9 in, 5 out]
    n241 = Read from Text File(file (use dialog)=w213) -> (text=w214:string)  [unwired: 3 in, 3 out]
    n242 = Read from Text File(file (use dialog)=w208) -> (text=w207:string)  [unwired: 3 in, 3 out]
    n243 = Spreadsheet String To Array(format string=w212, spreadsheet string=w214, array type (2D Dbl)=w212) -> (array=w215:string[][])  [unwired: 1 in]
    n244 = Spreadsheet String To Array(delimiter (Tab)="\\n", format string=w202, spreadsheet string=w207, array type (2D Dbl)=w202) -> (array=w206:string[][])
    n245 = Index Array(array=w215, index (col)=0 ("index")) -> (element=w209:string[])  [unwired: 1 in]
    "Usuarios 2" <- w209
    n246 = Index Array "Index Array"(array=w209) -> ()  [unwired: 2 in, 2 out]
    n247 = Array Size(array=w209) -> (size(s)=w216:i32)
    "element 3" <- w216
    n248 = Index Array(array=w206, index (col)=1 ("disabled index (col)")) -> ()  [unwired: 1 in, 1 out]
    n249 = for {
      N: w216 -> [_]
      n250 = local read "Usuarios 2"() -> (w229:string[])
      n251 = local read "Nuevo usuario 2"() -> (w227:string)
      n252 = Index Array(array=w229) -> (element=w228:string)  [unwired: 1 in]
      n253 = Equal?(x=w228, y=w227) -> (x = y?=w226:bool)
      n254 = case shown="True" w226 {
        frame False {
        }
        frame True {
        }
      }
    }
    n255 = Index Array(array=w206, index (col)=0 ("index")) -> (element=w205:string[])  [unwired: 1 in]
    n256 = local write "Usuarios y contraseñas 2"(w205) -> ()
  }
  n257 = Close File(refnum=w7, error in=w10) -> (error out=w9:errorcluster)  [unwired: 1 out]
  n258 = Close File(refnum=w18, error in=w21) -> (error out=w20:errorcluster)  [unwired: 1 out]
  n259 = call <vilib>:"Simple Error Handler.vi"("error in (no error)"=w9) -> ()  [unwired: 4 in, 5 out]
  n260 = call <vilib>:"Simple Error Handler.vi"("error in (no error)"=w20) -> ()  [unwired: 4 in, 5 out]
  "Tab Control" <- T1."Log" ("Tab Control")
  "Tab Control 2" <- T1."Log" ("Tab Control")
